vi "REACTOR_PARSE_SET_VALVULA.vi"(11 "String":string="VALVULA: 1, TEMPERATURA 35.0C") -> (1 "Temperatura (C)":dbl=1.0, 2 "VALVULA 1":bool=TRUE)   [LabVIEW 2017]
panel:
  # "VALVULA: 1, TEMPERATURA 35.0C"
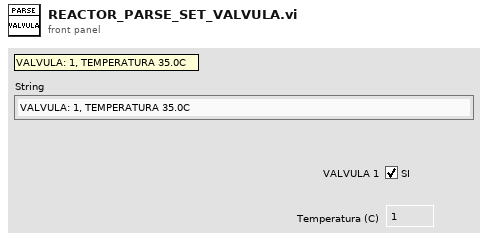
[diagram p1: front panel]
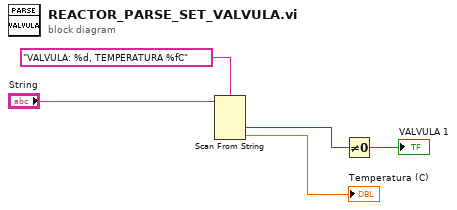
[diagram p0: block diagram]
diagram:
  n1 = Scan From String(format string="VALVULA: %d, TEMPERATURA %fC", input string="String") -> (output 1=w4:i32, output 2=→"Temperatura (C)":dbl)  [unwired: 4 in, 3 out]
  n2 = Not Equal To 0?(x=w4) -> (x != 0?=→"VALVULA 1":bool)
